vi "Read Strings.vi"(8 "error in (no error)":errorcluster, 11 "Concatenate_STR in":refnum<class "Concatenate_STR.lvclass">) -> (0 "error out":errorcluster, 2 "Strings":refnum<class "Abs_Value.lvclass">[](array[class]), 3 "Concatenate_STR out":refnum<class "Concatenate_STR.lvclass">)   [LabVIEW 2021, in "Concatenate_STR.lvclass"]
uses:
  Concatenate_STR.lvclass
  Abs_Types/Value/Abs_Value.lvclass
  Concatenate_STR.lvclass/Concatenate_STR.ctl
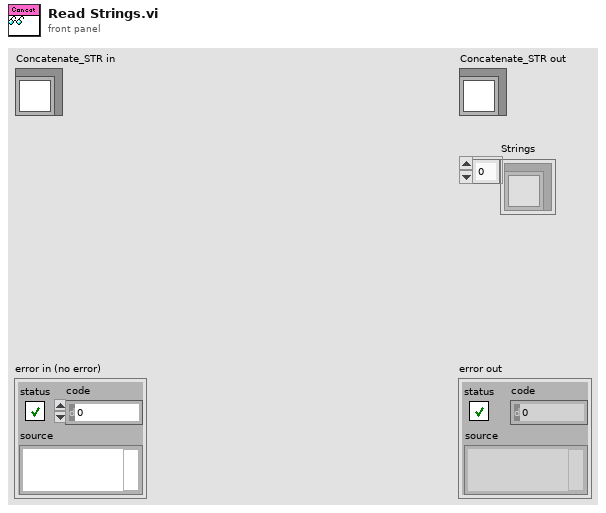
[diagram p1: front panel]
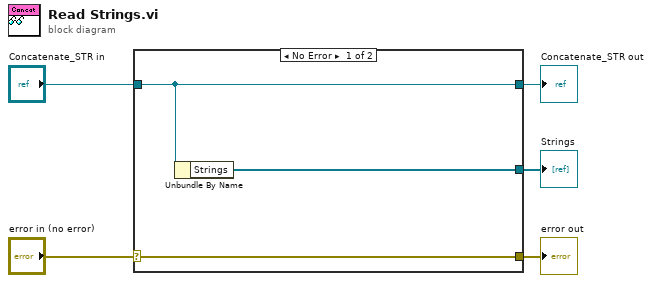
[diagram p0: block diagram]
diagram:
  n1 = case shown="No Error" "error in (no error)" {
    selector: "error in (no error)" -> [w8 w9]
    tunnel: [w8 w9] -> w4
    tunnel: [w7 w10] -> w2
    tunnel: "Concatenate_STR in" -> [w7 w10]
    tunnel: [w6 _] -> w1
    frame No Error {
      n2 = Unbundle By Name(w7) -> ("Strings"=w6:refnum<class "Abs_Value.lvclass">[])
    }
    frame Error {
    }
  }
  "error out" <- w4
  "Concatenate_STR out" <- w2
  "Strings" <- w1
